vi "WFS Get Highspeed Windows.vi"(8 "error in (no error)":errorcluster {"code" format="%.0x"}, 11 "instrument handle":refnum<visa-resource-name>) -> (0 "error out":errorcluster {"code" format="%.0x"}, 1 "Window Count Y":i32, 2 "Window Count X":i32, 3 "instrument handle out":refnum<visa-resource-name>, 4 "Window Size X":i32, 5 "Window Size Y":i32, 6 "Window Startpos X":i32[](array[numeric]), 7 "Window Startpos Y":i32[](array[numeric]))   [LabVIEW 2020]
doc: "This VI returns data of the spot detection windows valid in Highspeed Mode. Window size and positions depend on options passed to WFS Set Highspeed Mode.vi().\n\nNote: This VI is only available when Highspeed Mode is activated!"
uses:
  WFS_32.dll
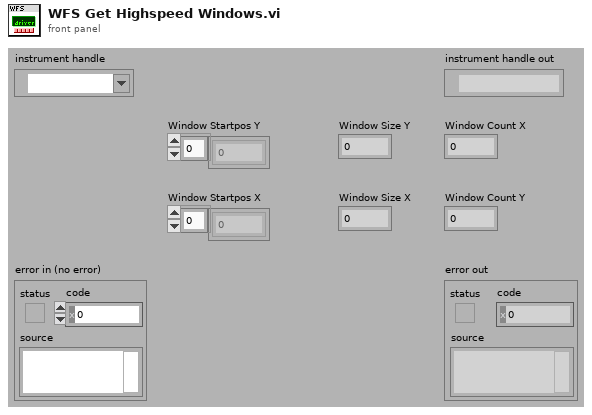
[diagram p1: front panel]
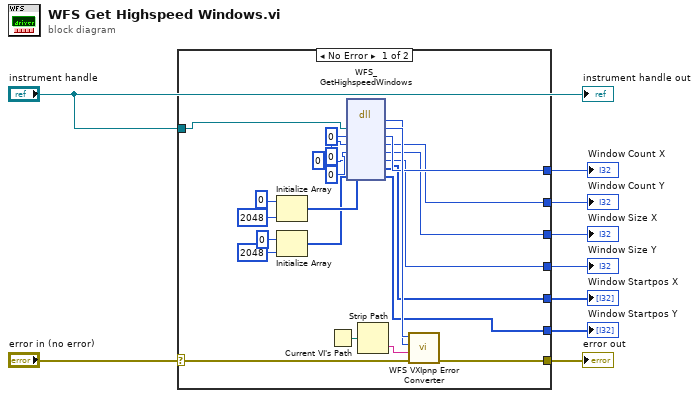
[diagram p0: block diagram]
diagram:
  n1 = case shown="No Error" "error in (no error)" {
    selector: "error in (no error)" -> [w27 w33]
    tunnel: [w26 w33] -> w9
    tunnel: "instrument handle" -> [w31 _]
    tunnel: [w24 _] -> w6
    tunnel: [w22 _] -> w5
    tunnel: [w20 _] -> w4
    tunnel: [w18 _] -> w3
    tunnel: [w14 _] -> w2
    tunnel: [w10 _] -> w1
    frame No Error {
      n2 = Initialize Array(0 ("element"), 2048 ("dimension size")) -> (w17:i32[])
      n3 = Initialize Array(0 ("element"), 2048 ("dimension size")) -> (w13:i32[])
      n4 = Current VI's Path() -> (path=w32:path)
      n5 = dll-call lib="WFS_*.*" fn="WFS_GetHighspeedWindows"("Instrument Handle"=w31, "Window Count X"=0, "Window Count Y"=0, "Window Size X"=0, "Window Size Y"=0, "Window Startpos X"=w17, "Window Startpos Y"=w13) -> (w29:i32, "Instrument Handle"=w30:u32, "Window Count X"=w24:i32, "Window Count Y"=w22:i32, "Window Size X"=w20:i32, "Window Size Y"=w18:i32, "Window Startpos X"=w14:i32[], "Window Startpos Y"=w10:i32[])  [unwired: 3 in, 2 out]
      n6 = Strip Path(path=w32) -> (name=w28:string)  [unwired: 1 out]
      n7 = call "WFS VXIpnp Error Converter.vi"("error in (no error)"=w27, "Name Of VI (\"\")"=w28, "CVI Error Code (0)"=w29, "instrument handle"=w30) -> ("error out"=w26:errorcluster)  [unwired: 6 in, 1 out]
    }
    frame Error {
    }
  }
  "error out" <- w9
  "Window Count X" <- w6
  "Window Count Y" <- w5
  "Window Size X" <- w4
  "Window Size Y" <- w3
  "Window Startpos X" <- w2
  "Window Startpos Y" <- w1
  "instrument handle out" <- "instrument handle"
